vi "Case Scripter.vi"() -> ()   [LabVIEW 2019]
uses:
  Source/VI Scripting Utilities/VI Scripting Utilities.lvlib
panel:
  out "error IO":errorcluster
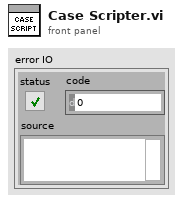
[diagram p1: front panel]
types:
  T1 = enum32{"Strict", "Allow Wires Under Labels", "Allow Wires Under Lead Nodes", "Allow Wires Under Wide Blocks"}
  T2 = enum32{"Left", "Right", "Hybrid", "Center", "Gravity"}
  T3 = cluster{"Alignment":enum32{"Left", "Right", "Hybrid", "Center", "Gravity"}, "Rules":enum32{"Strict", "Allow Wires Under Labels", "Allow Wires Under Lead Nodes", "Allow Wires Under Wide Blocks"}, "Max Heuristic Iterations":u32, "Max Simplex Iterations":u32, "Block Padding":cluster{"Horizontal":i32, "Vertical":i32}, "Wire Padding":cluster{"Horizontal":i32, "Vertical":i32}, "Auto-Tune by Topology":bool, "Fine-Tune Y Positions":bool, "Align All Controls on Left":bool, "Align All Indicators on Right":bool, "Use Array Dimension Heuristics":bool}
  T4 = typedef "LVPointTypeDef.ctl" = cluster{"Horizontal":i16, "Vertical":i16}
  T5 = typedef "LVBoundsTypeDef.ctl" = cluster{"Width":u32, "Height":u32}
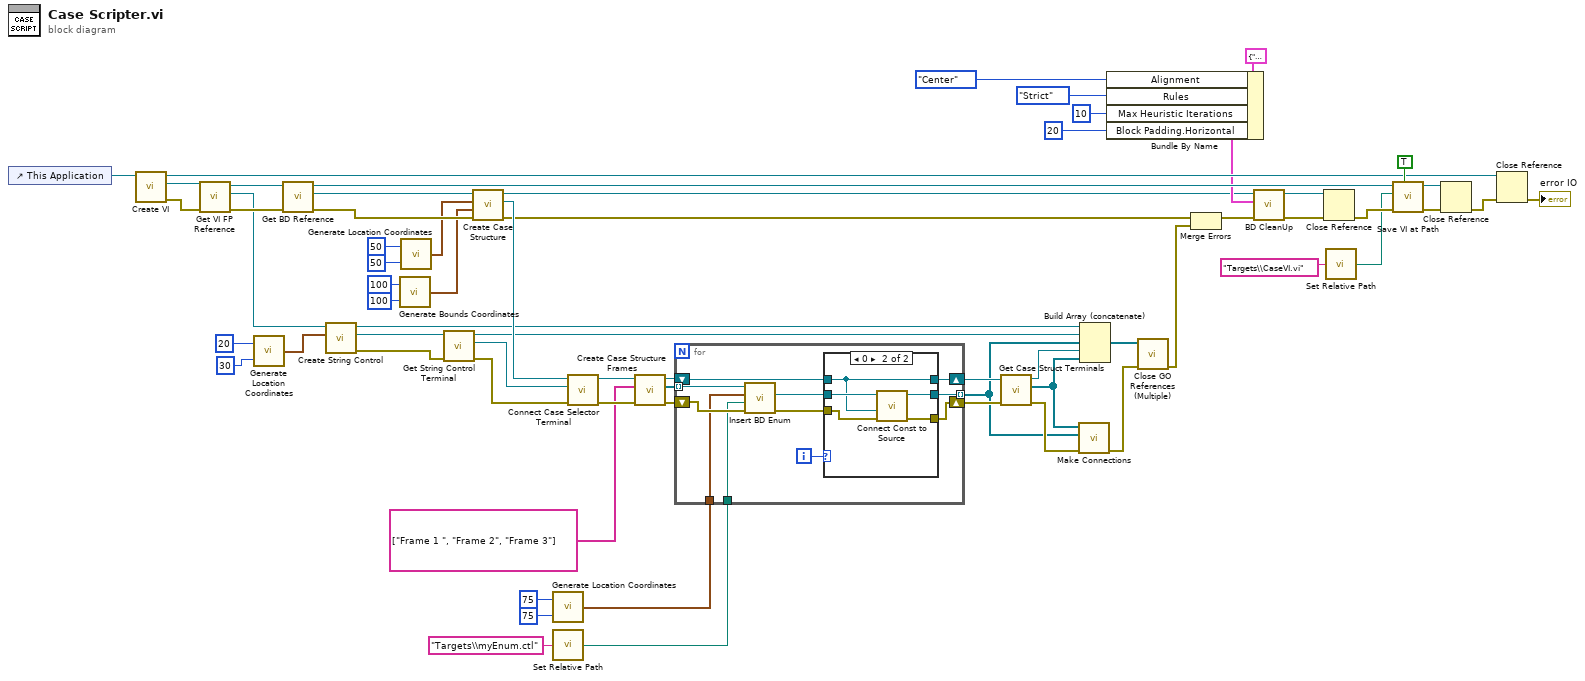
[diagram p0: block diagram]
diagram:
  n1 = control-ref of="This Application"() -> (w65:refnum<vi>)
  n2 = call "Create VI.vi"("Application in"=w65) -> ("error out"=w61:errorcluster, "New VI"=w62:refnum<vi>, "Application out"=w47:refnum<vi>)  [unwired: 8 in]
  n3 = call "Get VI FP Reference.vi"("error in (no error)"=w61, "VI in"=w62) -> ("error out"=w63:errorcluster, "Front Panel"=w58:refnum<vi>, "VI out"=w64:refnum<vi>)  [unwired: 7 in]
  n4 = call "Generate Location Coordinates.vi"("Vertical"=i16 30 ("Horizontal"), "Horizontal"=i16 20) -> ("Location out"=w1:T4)
  n5 = call "Get BD Reference.vi"("error in"=w63, "VI in"=w64) -> ("error out"=w59:errorcluster, "Block Diagram"=w60:refnum<vi>, "VI out"=w26:refnum<vi>)  [unwired: 7 in]
  n6 = call "Create String Control.vi"("location"=w1, "Front Panel in"=w58) -> ("error out"=w56:errorcluster, "String Control"=w57:refnum<vi>, "Front Panel out"=w14:refnum<vi>)  [unwired: 7 in]
  n7 = call "Generate Bounds Coordinates.vi"("Height"=u32 100, "Width"=u32 100) -> ("bounds"=w40:T5)
  n8 = call "Generate Location Coordinates.vi"("Vertical"=i16 50 ("Horizontal"), "Horizontal"=i16 50) -> ("Location out"=w41:T4)
  n9 = call "Get String Control Terminal.vi"("error in (no error)"=w56, "String Control in"=w57) -> ("error out"=w54:errorcluster, "Terminal"=w55:refnum<vi>, "String Control out"=w15:refnum<vi>)  [unwired: 7 in]
  n10 = call "Create Case Structure.vi"("error in (no error)"=w59, "bounds"=w40, "location"=w41, "Block Diagram in"=w60) -> ("error out"=w28:errorcluster, "Case Structure out"=w53:refnum<vi>, "Block Diagram out"=w7:refnum<vi>)  [unwired: 5 in]
  n11 = call "Generate Location Coordinates.vi"("Vertical"=i16 75 ("Horizontal"), "Horizontal"=i16 75) -> ("Location out"=w30:T4)
  n12 = call "Set Relative Path.vi"("App Relative Path"="Targets\\myEnum.ctl") -> ("Full Path"=w31:path)
  n13 = call "Connect Case Selector Terminal.vi"("error in (no error)"=w54, "Wire Source"=w55, "Case Structure in"=w53) -> ("error IO"=w51:errorcluster, "Case Structure out"=w52:refnum<vi>)  [unwired: 7 in]
  n14 = call "Create Case Structure Frames.vi"("error in (no error)"=w51, "Frame Names"=string[] ["Frame 1 ", "Frame 2", "Frame 3"], "CaseStructure in"=w52) -> ("error out"=w33:errorcluster, "Case Frames[]"=w32:refnum<vi>[], "CaseStructure out"=w34:refnum<vi>)  [unwired: 6 in]
  n15 = for {
    tunnel: w32 -> [w76] mode=indexing
    shift-right: [w69] -> w18
    shift-left: w34 -> [w70]
    tunnel: w31 -> [w74]
    tunnel: w30 -> [w73]
    shift-right: [w66] -> w17
    shift-left: w33 -> [w75]
    tunnel: [w67] -> w13 mode=indexing
    i -> [w72]
    n16 = call "Insert BD Enum.vi"("error in (no error)"=w75, "path"=w74, "BD Location"=w73, "Owner  in"=w76) -> ("error out"=w68:errorcluster, "Enum out"=w71:refnum<vi>)  [unwired: 5 in, 1 out]
    n17 = case shown="0" w72 {
      tunnel: w71 -> [w77 w84]
      tunnel: w70 -> [w79 w83]
      tunnel: [w79 w83] -> w69
      tunnel: w68 -> [w78 w82]
      tunnel: [w78 w81] -> w66
      tunnel: [w77 w80] -> w67
      frame 1, Default {
      }
      frame 0 {
        n18 = call "Connect Const to Source.vi"("Error In"=w82, "Source"=w83, "Const in"=w84) -> ("Error Out"=w81:errorcluster, "Const out"=w80:refnum<vi>)  [unwired: 7 in]
      }
    }
  }
  n19 = call "Get Case Struct Terminals.vi"("Error In"=w17, "Case Structure in"=w18) -> ("Error Out"=w16:errorcluster, "Tunnels[]"=w11:refnum<vi>[], "Case Structure out"=w12:refnum<vi>)  [unwired: 7 in]
  n20 = call "Make Connections.vi"("error in (no error)"=w16, "Enums in"=w13, "Tunnel in"=w11) -> ("error out"=w9:errorcluster)  [unwired: 8 in]
  n21 = Build Array (concatenate)(w14, w15, w13, w12, w11) -> (w10:refnum<vi>[])
  n22 = Bundle By Name(cluster=T3 {"Alignment"=enum."Left", "Rules"=enum."Strict", "Max Heuristic Iterations"=0, "Max Simplex Iterations"=0, "Block Padding"={"Horizontal"=0, "Vertical"=0}, "Wire Padding"={"Horizontal"=0, "Vertical"=0}, "Auto-Tune by Topology"=FALSE, "Fine-Tune Y Positions"=FALSE, "Align All Controls on Left"=FALSE, "Align All Indicators on Right"=FALSE, "Use Array Dimension Heuristics"=FALSE} ("Clean Up Options"), "Alignment"=T2."Center", "Rules"=T1."Strict", "Max Heuristic Iterations"=u32 10, "Block Padding.Horizontal"=20) -> (w19:T3)
  n23 = call "Close GO References (Multiple).vi"("Error In"=w9, "References in"=w10) -> ("Error Out"=w8:errorcluster)  [unwired: 9 in]
  n24 = Merge Errors(w28, w8) -> (w29:errorcluster)
  n25 = call "BD CleanUp.vi"("error in (no error)"=w29, "Clean Up Options"=w19, "Block Diagram in"=w7) -> ("error out"=w44:errorcluster, "Block Diagram out"=w45:refnum<vi>)  [unwired: 7 in]
  n26 = Close Reference(reference=w45, error in (no error)=w44) -> (error out=w27:errorcluster)
  n27 = call "Set Relative Path.vi"("App Relative Path"="Targets\\CaseVI.vi" ("name or relative path")) -> ("Full Path"=w25:path)
  n28 = call "Save VI at Path.vi"("Override Existing? (T)"=TRUE, "error in (no error)"=w27, "Path"=w25, "VI in"=w26) -> ("error out"=w6:errorcluster, "VI out"=w5:refnum<vi>)  [unwired: 6 in]
  n29 = Close Reference(reference=w5, error in (no error)=w6) -> (error out=w4:errorcluster)
  n30 = Close Reference(reference=w47, error in (no error)=w4) -> (error out=→"error IO":errorcluster)
